vi "Open.vi"(8 "error in (no error)":errorcluster, 11 "HslCommunication:MelsecFxLinksOverTcp in":refnum<class "MelsecFxLinksOverTcp.lvclass">) -> (0 "error out":errorcluster, 3 "HslCommunication:MelsecFxLinksOverTcp out":refnum<class "MelsecFxLinksOverTcp.lvclass">)   [LabVIEW 2020, in "HslCommunication.lvlib" / "MelsecFxLinksOverTcp.lvclass"]
uses:
  MelsecFxLinksOverTcp.lvclass
  MelsecFxLinksOverTcp.lvclass/MelsecFxLinksOverTcp.ctl
  E:/Git/Libraries/develop/HslCommunication/_Dependenciecs/HslCommunication.dll
  _Dependenciecs/HslCommunication.dll
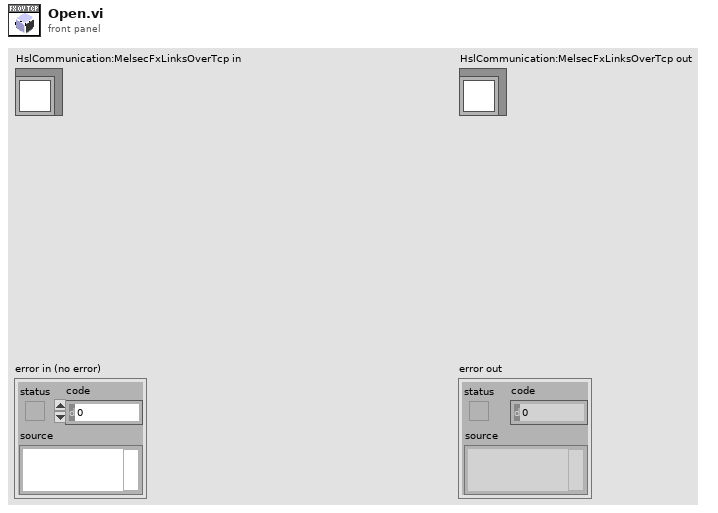
[diagram p1: front panel]
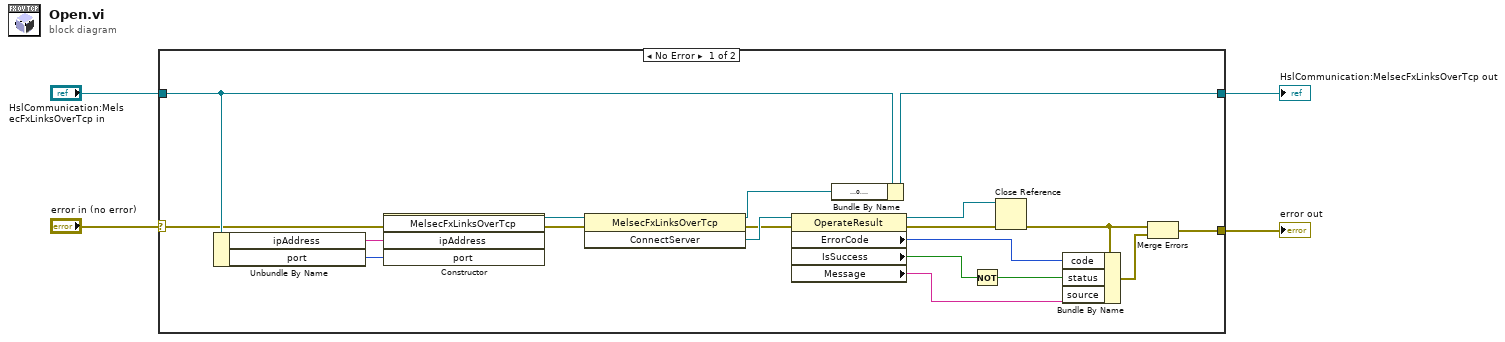
[diagram p0: block diagram]
diagram:
  n1 = case shown="No Error" "error in (no error)" {
    selector: "error in (no error)" -> [w6 w25]
    tunnel: "HslCommunication:MelsecFxLinksOverTcp in" -> [w12 w24]
    tunnel: [w23 w24] -> w1
    tunnel: [w18 w25] -> w2
    frame No Error {
      n2 = Unbundle By Name(w12) -> ("ipAddress"=w10:string, "port"=w9:i32)
      n3 = constructor class="MelsecFxLinksOverTcp"(error in=w6, "ipAddress"=w10, "port"=w9) -> (reference out=w8:refnum<k24>, error out=w7:errorcluster)  [unwired: 2 in, 3 out]
      n4 = invoke class="MelsecFxLinksOverTcp" method="ConnectServer"(reference=w8, error in=w7) -> (reference out=w5:refnum<k24>, error out=w13:errorcluster, "ConnectServer"=w14:refnum<k24>)  [unwired: 1 in]
      n5 = property class="OperateResult"(reference=w14, error in=w13) -> (reference out=w17:refnum<k24>, error out=w16:errorcluster, "ErrorCode"=w21:i32, "IsSuccess"=w15:bool, "Message"=w19:string)
      n6 = Bundle By Name(cluster=w12, "reference"=w5) -> (w23:refnum<class "MelsecFxLinksOverTcp.lvclass">)
      n7 = Not(x=w15) -> (.not. x?=w20:bool)
      n8 = Close Reference(reference=w17, error in (no error)=w16) -> (error out=w11:errorcluster)
      n9 = Bundle By Name(cluster=w11, "code"=w21, "status"=w20, "source"=w19) -> (w22:errorcluster)
      n10 = Merge Errors(w11, w22) -> (w18:errorcluster)
    }
    frame Error {
    }
  }
  "error out" <- w2
  "HslCommunication:MelsecFxLinksOverTcp out" <- w1
